vi "Align to 8-byte Boundary.vi"(11 "pointer":u32 format="%08x") -> (3 "aligned pointer":u32 format="%08x")   [LabVIEW 2016, in "GE 5565PIORC Old.lvclass"]
uses:
  GE 5565PIORC Old.lvclass
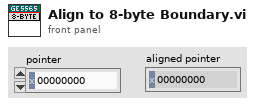
[diagram p1: front panel]
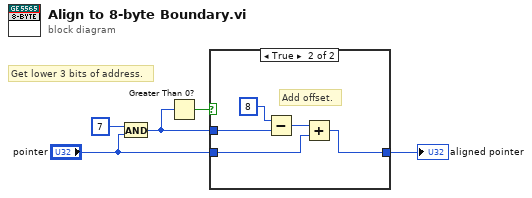
[diagram p0: block diagram]
diagram:
  # "Get lower 3 bits of address."
  n1 = And(x=u32 7, y="pointer") -> (x .and. y?=w2:u32)
  n2 = Greater Than 0?(x=w2) -> (x > 0?=w1:bool)
  n3 = case shown="True" w1 {
    tunnel: [w6 w11] -> w5
    tunnel: w2 -> [_ w9]
    tunnel: "pointer" -> [w6 w8]
    frame False {
      # "Already aligned."
    }
    frame True {
      # "Add offset."
      n4 = Subtract(x=u32 8, y=w9) -> (x-y=w10:u32)
      n5 = Add(x=w10, y=w8) -> (x+y=w11:u32)
    }
  }
  "aligned pointer" <- w5
